vi "Synchronize Palette with Directory.vi"() -> ()   [LabVIEW 2015]
panel:
  out "error out":errorcluster
  in  "error in (no error)":errorcluster
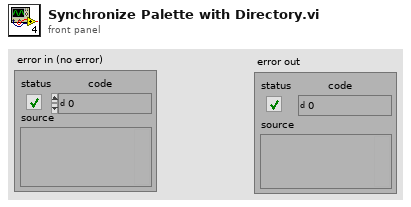
[diagram p1: front panel]
types:
  T1 = typedef "Palette Menu.lvlib/Palette Data.ctl" = cluster{"display name":string, "view format":T2, "palette width":i16, "items":T3, "256 color icon":picture, "B&W color icon":picture, "help information":T5, "palette description":string, "synchronize information":T6}
  T2 = typedef "Palette Menu.lvlib/View Format.ctl" = u16
  T3 = typedef "Palette Menu.lvlib/Items.ctl" = T4[]
  T4 = typedef "Palette Menu.lvlib/Item.ctl" = cluster{"item path":path, "library path (.lvlib)":path, "use default lvlib palette":bool, "short name":string, "place VI contents":bool, "hide synchronized item":bool, "reserve spot for synch item":bool, "configure when placing VI contents":bool}
  T5 = typedef "Palette Menu.lvlib/Help Info.ctl" = cluster{"help tag":string, "help file path ":path}
  T6 = typedef "Palette Menu.lvlib/Synchronize Info.ctl" = cluster{"synchronize with directory":bool, "synchronize directory path":path}
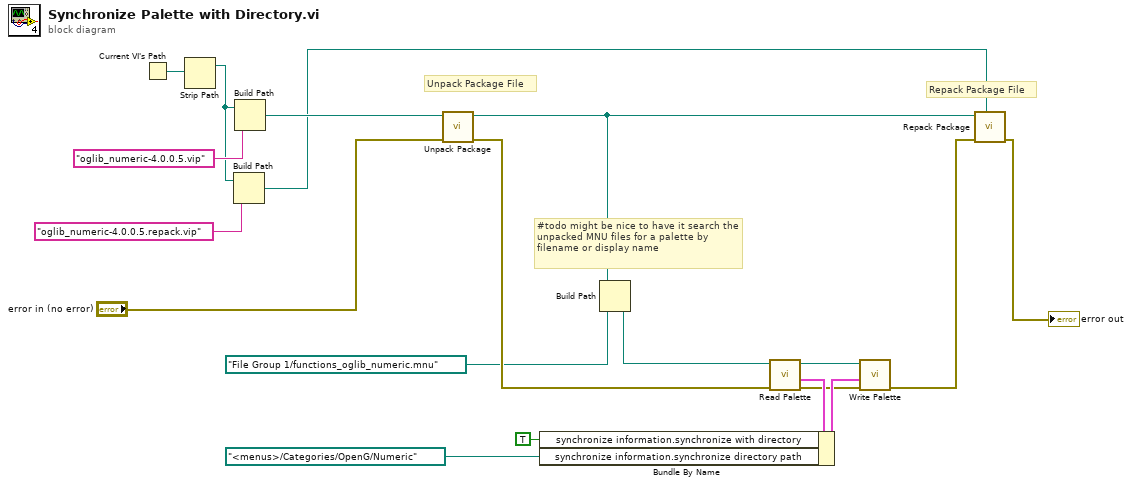
[diagram p0: block diagram]
diagram:
  # "Repack Package File"
  # "Unpack Package File"
  # "#todo might be nice to have it search the unpacked MNU files for a palette by filename or display name"
  n1 = Current VI's Path() -> (path=w19:path)
  n2 = Strip Path(path=w19) -> (stripped path=w15:path)  [unwired: 1 out]
  n3 = Build Path(base path=w15, name or relative path="oglib_numeric-4.0.0.5.repack.vip") -> (appended path=w1:path)
  n4 = Build Path(base path=w15, name or relative path="oglib_numeric-4.0.0.5.vip") -> (appended path=w17:path)
  n5 = call "Unpack Package.vi"("error in (no error)"="error in (no error)", "Package File"=w17) -> ("error out"=w11:errorcluster, "Unpacked Package Directory"=w2:path)  [unwired: 7 in, 1 out]
  n6 = Build Path(base path=w2, name or relative path=path "File Group 1/functions_oglib_numeric.mnu" ("Unpacked File")) -> (appended path=w3:path)
  n7 = call <vilib>:"Read Palette.vi"("error in (no error)"=w11, "palette path"=w3) -> ("error out"=w5:errorcluster, "palette data"=w8:T1, "duplicate palette path"=w9:path)  [unwired: 7 in]
  n8 = Bundle By Name(cluster=w8, "synchronize information.synchronize with directory"=TRUE, "synchronize information.synchronize directory path"=path "<menus>/Categories/OpenG/Numeric" ("Unpacked File")) -> (w7:T1)
  n9 = call <vilib>:"Write Palette.vi"("error in (no error)"=w5, "palette data"=w7, "palette path"=w9) -> ("error out"=w10:errorcluster)  [unwired: 8 in]
  n10 = call "Repack Package.vi"("Package File (\"\": use name of directory to repack)"=w1, "error in (no error)"=w10, "Directory to repack"=w2) -> ("error out"=→"error out":errorcluster)  [unwired: 8 in]
